vi "VHM-continiousDataSetHandler.vi"(8 "error in (no error)":errorcluster, 11 "VHM-VNA_Hardware_Manager in":refnum<class "VHM-VNA_Hardware_Manager.lvclass">) -> (0 "error out":errorcluster, 3 "VHM-VNA_Hardware_Manager out":refnum<class "VHM-VNA_Hardware_Manager.lvclass">)   [LabVIEW 2020, in "VHM-VNA_Hardware_Manager.lvlib" / "VHM-VNA_Hardware_Manager.lvclass"]
uses:
  VHM-VNA_Hardware_Manager.lvclass
  C:/Program Files (x86)/National Instruments/LabVIEW 2020/vi.lib/ActorFramework/Actor/Actor.lvclass
  VHM-VNA_Hardware_Manager.lvclass/VHM-VNA_Hardware_Manager.ctl
  VHM-VNA_Hardware_Manager Messages/VHM-getDataSet Msg/VHM-getDataSet Msg.lvclass
  C:/Program Files (x86)/National Instruments/LabVIEW 2020/vi.lib/ActorFramework/Message/Message.lvclass
  <vilib>/ActorFramework/Actor/Actor.lvclass/Actor.ctl
  <vilib>/ActorFramework/Message Enqueuer/Message Enqueuer.lvclass/Message Enqueuer.ctl
  <vilib>/ActorFramework/Message Enqueuer/Init from Existing Queue.vi
  <vilib>/ActorFramework/Message Enqueuer/Message Enqueuer.lvclass
  <vilib>/ActorFramework/Actor/Actor.lvclass
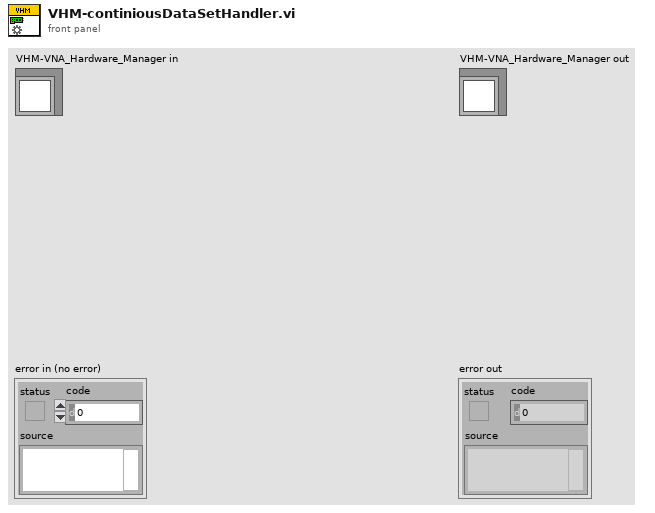
[diagram p1: front panel]
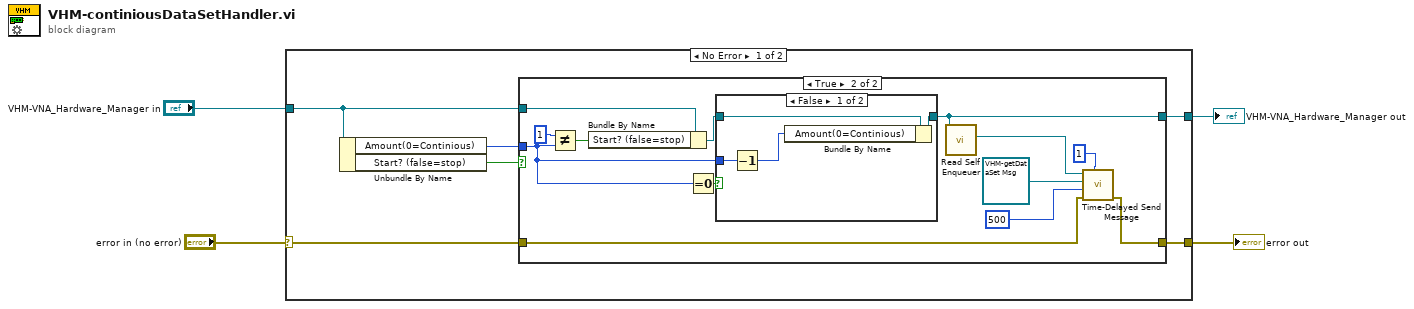
[diagram p0: block diagram]
diagram:
  n1 = case shown="No Error" "error in (no error)" {
    selector: "error in (no error)" -> [w6 w32]
    tunnel: [w5 w32] -> w3
    tunnel: [w9 w31] -> w1
    tunnel: "VHM-VNA_Hardware_Manager in" -> [w10 w31]
    frame No Error {
      n2 = Unbundle By Name(w10) -> ("Amount(0=Continious)"=w7:u8, "Start? (false=stop)"=w8:bool)
      n3 = case shown="True" w8 {
        tunnel: w10 -> [w12 w24]
        tunnel: [w12 w14] -> w9
        tunnel: w7 -> [_ w13]
        tunnel: w6 -> [w11 w18]
        tunnel: [w11 w17] -> w5
        frame False {
        }
        frame True {
          n4 = Not Equal?(x=u8 1, y=w13) -> (x != y?=w23:bool)
          n5 = Bundle By Name(cluster=w24, "Start? (false=stop)"=w23) -> (w15:refnum<class "VHM-VNA_Hardware_Manager.lvclass">)
          n6 = Equal To 0?(x=w13) -> (x = 0?=w16:bool)
          n7 = case shown="False" w16 {
            tunnel: w15 -> [w29 w30]
            tunnel: [w28 w30] -> w14
            tunnel: w13 -> [w27 _]
            frame False {
              n8 = Decrement(x=w27) -> (x-1=w26:u8)
              n9 = Bundle By Name(cluster=w29, "Amount(0=Continious)"=w26) -> (w28:refnum<class "VHM-VNA_Hardware_Manager.lvclass">)
            }
            frame True {
            }
          }
          n10 = call <vilib>:"Read Self Enqueuer.vi"("Actor"=w14) -> ("Self Enqueuer"=w20:refnum<class "Message Enqueuer.lvclass">)  [unwired: 10 in]
          n11 = call <vilib>:"Time-Delayed Send Message.vi"("# Copies (0 = infinite repeat)"=u32 1, "error in (no error)"=w18, "Milliseconds To Wait"=500, "Message"=refnum<class "VHM-getDataSet Msg.lvclass"> refnum ("VHM-VNA_Hardware_Manager.lvlib:VHM-getDataSet Msg.lvclass"), "Message Enqueuer"=w20) -> ("error out"=w17:errorcluster)  [unwired: 5 in, 1 out]
        }
      }
    }
    frame Error {
    }
  }
  "error out" <- w3
  "VHM-VNA_Hardware_Manager out" <- w1
